vi "Is Open.vi"(8 "error in (no error)":errorcluster, 11 "Websocket Server in":refnum<class "Websocket Server.lvclass">) -> (0 "error out":errorcluster, 2 "Is Open":bool, 3 "Websocket Server out":refnum<class "Websocket Server.lvclass">)   [LabVIEW 2020, in "Stream-Websocket.lvlib" / "Websocket Server.lvclass"]
uses:
  Websocket Server.lvclass
  Websocket Server.lvclass/Websocket Server.ctl
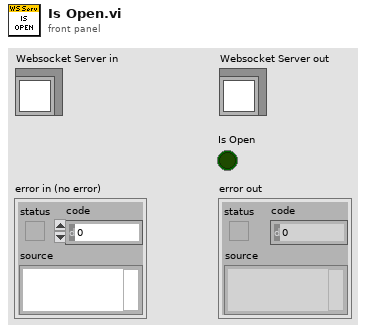
[diagram p1: front panel]
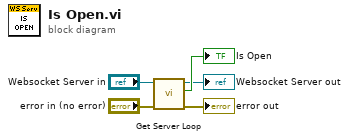
[diagram p0: block diagram]
diagram:
  n1 = call "Get Server Loop.vi"("error in (no error)"="error in (no error)", "Websocket Server in"="Websocket Server in") -> ("error out"=→"error out":errorcluster, "Server Loop"=→"Is Open":bool, "Websocket Server out"=→"Websocket Server out":refnum<class "Websocket Server.lvclass">)  [unwired: 7 in]
